vi "3.4.1-Battery Voltage Conversion.vi"(1 "Input":fxp<+/-,16,5>) -> (0 "Output":dbl)   [LabVIEW 2010]
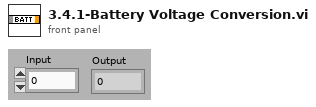
[diagram p1: front panel]
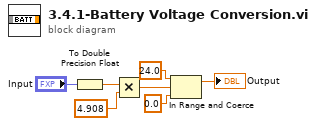
[diagram p0: block diagram]
diagram:
  n1 = To Double Precision Float(number="Input") -> (double precision float=w6:dbl)
  n2 = Multiply(x=w6, y=4.908) -> (x*y=w4:dbl)
  n3 = In Range and Coerce(upper limit=24.0, x=w4, lower limit=0.0) -> (coerced(x)=→"Output":dbl)  [unwired: 1 out]
